vi "Calculate N Cubes.vi"(8 "error in (no error)":errorcluster, 11 "Cubes in":refnum<class "Cubes.lvclass">) -> (0 "error out":errorcluster, 2 "N Cubes":i64, 3 "Cubes out":refnum<class "Cubes.lvclass">)   [LabVIEW 2019, in "22.lvlib" / "Cubes.lvclass"]
uses:
  Cubes.lvclass
  Cubes.lvclass/Cubes.ctl
  Cube/Cube.lvclass
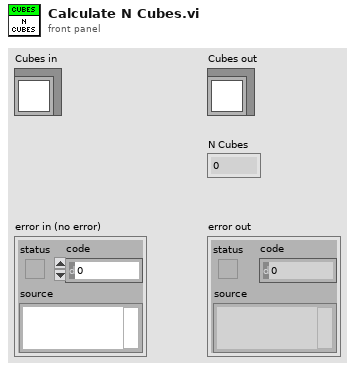
[diagram p1: front panel]
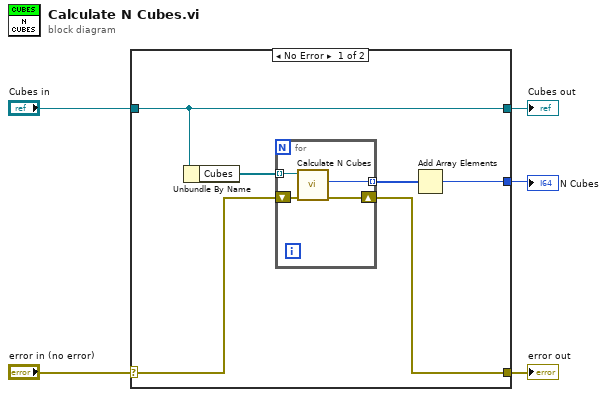
[diagram p0: block diagram]
diagram:
  n1 = case shown="No Error" "error in (no error)" {
    selector: "error in (no error)" -> [w9 w17]
    tunnel: [w8 w17] -> w4
    tunnel: [w11 w16] -> w2
    tunnel: "Cubes in" -> [w11 w16]
    tunnel: [w6 _] -> w1
    frame No Error {
      n2 = Unbundle By Name(w11) -> ("Cubes"=w10:refnum<class "Cube.lvclass">[])
      n3 = for {
        tunnel: w10 -> [w15] mode=indexing
        tunnel: [w14] -> w7 mode=indexing
        shift-right: [w12] -> w8
        shift-left: w9 -> [w13]
        n4 = call-dynamic "Calculate N Cubes.vi"("error in (no error)"=w13, "Cube in"=w15) -> ("error out"=w12:errorcluster, "N Cubes"=w14:i64)  [unwired: 7 in, 1 out]
      }
      n5 = Add Array Elements(numeric array=w7) -> (sum=w6:i64)
    }
    frame Error {
    }
  }
  "error out" <- w4
  "Cubes out" <- w2
  "N Cubes" <- w1
